vi "template.vi"() -> ()   [LabVIEW 2018]
uses:
  <vilib>/Analysis/1siggen.llb/Ramp Pattern by Samples.vi
  <vilib>/Analysis/NI_AALBase.lvlib
panel:
  out "Sorted Array":variant[](array[variant])
  out "Sorted Keys":dbl[](array[numeric])
  in  "Keys":dbl[](array[numeric])
  in  "Array":variant[](array[variant])
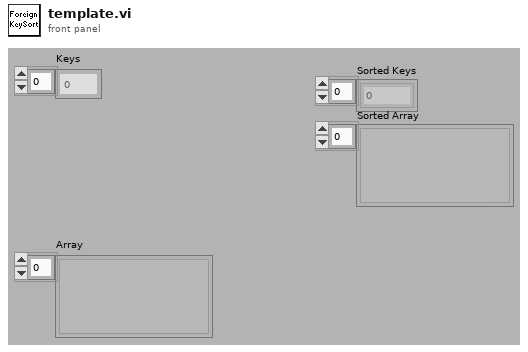
[diagram p1: front panel]
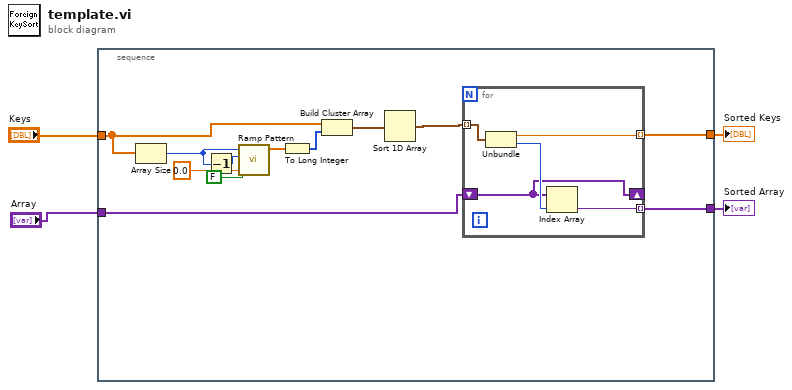
[diagram p0: block diagram]
diagram:
  n1 = stacked-sequence {
    tunnel: "Keys" -> [w10]
    tunnel: "Array" -> [w7]
    tunnel: [w6] -> w2
    tunnel: [w5] -> w1
    frame #0 {
      n2 = Array Size(array=w10) -> (size(s)=w15:i32)
      n3 = Decrement(x=w15) -> (x-1=w16:i32)
      n4 = call-poly <vilib>:"Ramp Pattern.vi"("exclude end?"=FALSE, "start"=0.0, "end"=w16, "samples"=w15) -> ("Ramp Pattern"=w12:dbl[])  [unwired: 6 in, 1 out]
      n5 = To Long Integer(number=w12) -> (32bit integer=w11:i32[])
      n6 = Build Cluster Array(w10, w11) -> (w9:cluster{"Numeric":dbl, i32}[])
      n7 = Sort 1D Array(array=w9) -> (sorted array=w8:cluster{"Numeric":dbl, i32}[])
      n8 = for {
        tunnel: w8 -> [w21] mode=indexing
        shift-right: [w18] -> _
        shift-left: w7 -> [w18]
        tunnel: [w19] -> w6 mode=indexing
        tunnel: [w17] -> w5 mode=indexing
        n9 = Unbundle(w21) -> ("Numeric"=w19:dbl, w20:i32)
        n10 = Index Array(array=w18, index=w20) -> (element=w17:variant)
      }
    }
  }
  "Sorted Keys" <- w2
  "Sorted Array" <- w1
